vi "Fakedata Integration Test.vi"() -> ()   [LabVIEW 2023]
panel:
  out "Rows Detected":i32
  out "Dens":dbl[](array[numeric])
  out "Temp":dbl[](array[numeric])
  out "Pressure":dbl[](array[numeric])
  out "Time":dbl[](array[numeric]) format="%#.8f"
  in  "Rows to Init":i32
  # "INCOMING ARRAYS"
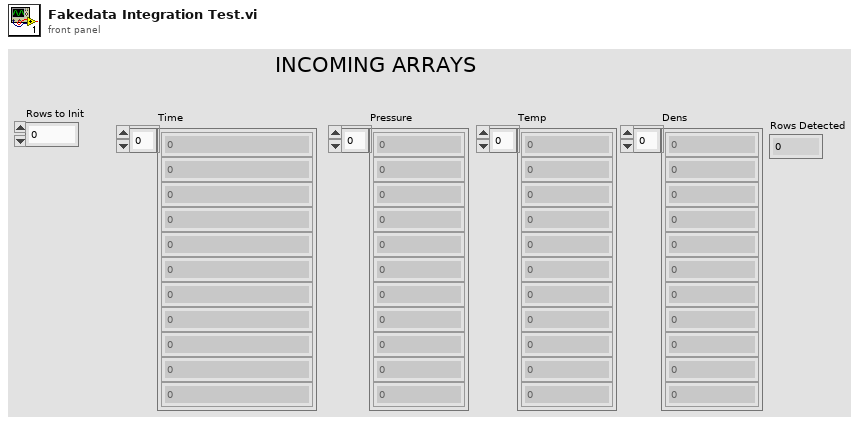
[diagram p1: front panel]
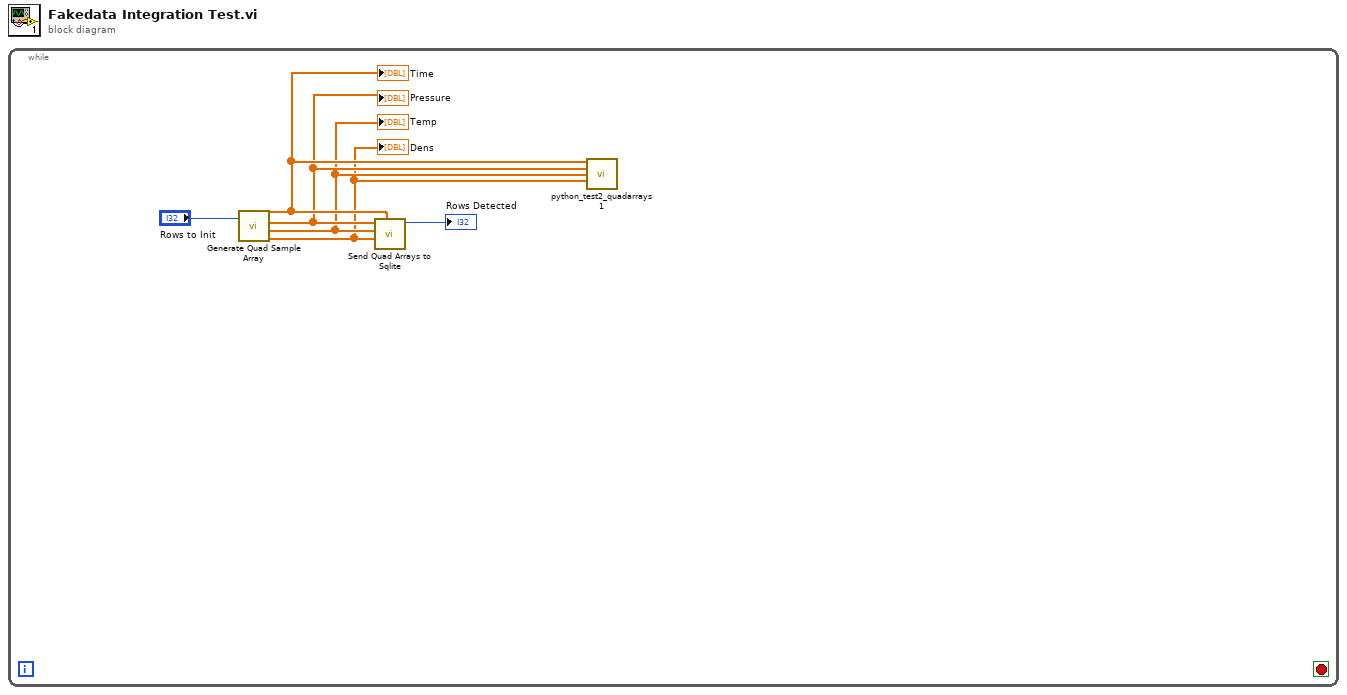
[diagram p0: block diagram]
diagram:
  n1 = while {
    stop <- _ stop-if-true
    n2 = call "Generate Quad Sample Array.vi"("Rows to Init"="Rows to Init") -> ("TIME Array"=w4:dbl[], "PRESS Array"=w3:dbl[], "TEMP Array"=w2:dbl[], "DENS Array"=w1:dbl[])  [unwired: 1 in]
    "Time" <- w4
    "Pressure" <- w3
    "Temp" <- w2
    "Dens" <- w1
    n3 = call "Send Quad Arrays to Sqlite.vi"("TIME 1D Array REAL"=w4, "DENS 1D Array REAL"=w1, "TEMP 1D Array REAL"=w2, "PRESSURE 1D Array REAL"=w3) -> ("Rows (Samples) Detected in input array"=→"Rows Detected":i32)  [unwired: 6 in, 1 out]
    n4 = call "python_test2_quadarrays 1.vi"("Time Array"=w4, "Press Array"=w3, "Temp Array"=w2, "Dens Array"=w1) -> ()  [unwired: 10 in, 2 out]
  }
